vi "testAo8b.vi"() -> ()   [LabVIEW 2011, in "run.lvlib"]
uses:
  Hal/testing/run.lvlib
  <vilib>/Utility/error.llb/DialogType.ctl
  <vilib>/DAQmx/write.llb/DAQmx Write (Analog 2D DBL NChan NSamp).vi
  <vilib>/DAQmx/create/channels.llb/DAQmx Create Channel (AO-Voltage-Basic).vi
  <vilib>/DAQmx/configure/timing.llb/DAQmx Timing (Sample Clock).vi
  <vilib>/DAQmx/miscellaneous.llb/DAQmx Fill In Error Info.vi
  Program Files/National Instruments/LabVIEW 2011/resource/objmgr/daqmx.rc
panel:
  out "CurrWritePos":dbl
  out "TotalSampPerChanGenerated":dbl
  out "number of samples written per channel":u32
  in  "Clock Source":tag="/Ao8b/PFI8"
  in  "stop":bool
  in  "Data":dbl[][](array[numeric])=[[0.0, -0.00465, -0.00465, -0.00465, -0.00465, -0.00465, -0.00465, -0.00423429, -0.00423429, -0.00423429, -0.00423429, -0.00423429, -0.00381858, -0.00381858, -0.00381858, -0.00381858, -0.00381858, -0.00381858, -0.0034028699999999997, -0.0034028699999999997, -0.0034028699999999997, -0.0034028699999999997, -0.0034028699999999997, -0.00298716, -0.00298716, -0.00298716, -0.00298716, -0.00298716, -0.00298716, -0.00257145, -0.00257145, -0.00257145, -0.00257145, -0.0021557399999999997, -0.0021557399999999997, -0.0021557399999999997, -0.0021557399999999997, -0.0021557399999999997, -0.0021557399999999997, -0.00174003, -0.00174003, -0.00174003, -0.00174003, -0.00174003, -0.00132432, -0.00132432, -0.00132432, -0.00132432, -0.00132432, -0.00132432, -0.0009086099999999998, -0.0009086099999999998, -0.0009086099999999998, -0.0009086099999999998, -0.0009086099999999998, -0.0004929000000000001, -0.0004929000000000001, -0.0004929000000000001, -0.0004929000000000001, -0.0004929000000000001, -0.0004929000000000001, -0.0004929000000000001, -0.0004929000000000001], [0.0, -0.01554, -0.01554, -0.01554, -0.0151700148, -0.0151700148, -0.0151700148, -0.0151700148, -0.0148000296, -0.0148000296, -0.0148000296, -0.0144300444, -0.0144300444, -0.0144300444, -0.014060059199999999, -0.014060059199999999, -0.014060059199999999, -0.014060059199999999, -0.014060059199999999, -0.013690074, -0.013690074, -0.0133200888, -0.0133200888, -0.0133200888, -0.0133200888, -0.012950103599999999, -0.012950103599999999, -0.012950103599999999, -0.0125801184, -0.0125801184, -0.0125801184, -0.0122101332, -0.0122101332, -0.0122101332, -0.011840148, -0.011840148, -0.011840148, -0.0114701628, -0.0114701628, -0.0114701628, -0.0114701628, -0.0111001776, -0.0111001776, -0.0107301924, -0.0107301924, -0.0107301924, -0.0107301924, -0.0107301924, -0.010360207199999999, -0.010360207199999999, -0.010360207199999999, -0.009990222, -0.009990222, -0.009990222, -0.0096202368, -0.0096202368, -0.0096202368, -0.0096202368, -0.009250251599999999, -0.009250251599999999, -0.0088802664, 0.0, 0.0], [0.0, -0.03996, -0.03996, -0.03996, -0.03996, -0.03996, -0.037739988, -0.037739988, -0.037739988, -0.037739988, -0.037739988, -0.035519976, -0.035519976, -0.035519976, -0.035519976, -0.035519976, -0.033299964, -0.033299964, -0.033299964, -0.033299964, -0.033299964, -0.031079952, -0.031079952, -0.031079952, -0.031079952, -0.031079952, -0.02885994, -0.02885994, -0.02885994, -0.02885994, -0.02885994, -0.026639928000000004, -0.026639928000000004, -0.026639928000000004, -0.026639928000000004, -0.026639928000000004, -0.024419916000000003, -0.024419916000000003, -0.024419916000000003, -0.024419916000000003, -0.024419916000000003, -0.022199904000000003, -0.022199904000000003, -0.022199904000000003, -0.022199904000000003, -0.022199904000000003, -0.019979892000000003, -0.019979892000000003, -0.019979892000000003, -0.019979892000000003, -0.019979892000000003, -0.017759880000000002, -0.017759880000000002, -0.017759880000000002, -0.017759880000000002, -0.017759880000000002, -0.015539868000000002, -0.015539868000000002, -0.015539868000000002, -0.015539868000000002, -0.015539868000000002, 0.0, 0.0], [0.0, -0.735, -0.735, -0.70673076, -0.70673076, -0.6784615199999999, -0.6784615199999999, -0.6784615199999999, -0.6784615199999999, -0.65019228, -0.62192304, -0.62192304, -0.62192304, -0.5936538, -0.5936538, -0.56538456, -0.56538456, -0.53711532, -0.53711532, -0.53711532, -0.50884608, -0.50884608, -0.48057684, -0.48057684, -0.4523076, -0.4523076, -0.4523076, -0.42403835999999995, -0.42403835999999995, -0.42403835999999995, -0.39576912, -0.36749988, -0.33923063999999997, -0.33923063999999997, -0.33923063999999997, -0.31096139999999994, -0.31096139999999994, -0.31096139999999994, -0.28269215999999997, -0.28269215999999997, -0.25442292, -0.25442292, -0.22615368000000002, -0.22615368000000002, -0.22615368000000002, -0.19788443999999994, -0.19788443999999994, -0.16961519999999997, -0.16961519999999997, -0.14134596, -0.14134596, -0.14134596, -0.11307671999999991, -0.08480747999999994, -0.08480747999999994, -0.08480747999999994, -0.08480747999999994, -0.05653823999999996, -0.05653823999999996, -0.02826899999999999, -0.02826899999999999, 0.0, 0.0]]
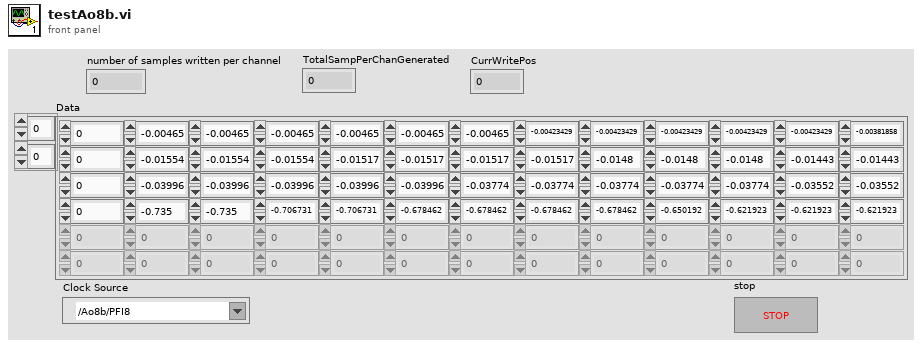
[diagram p1: front panel]
types:
  T1 = typedef "DialogType.ctl" = u16
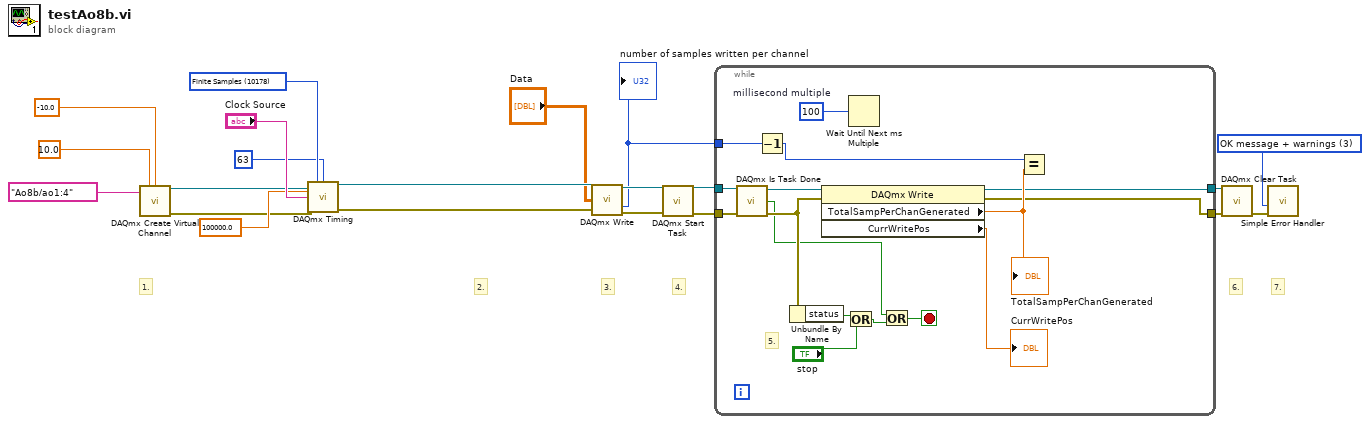
[diagram p0: block diagram]
diagram:
  w11 = T1 3 items=["no dialog", "OK message", "continue or stop message", "OK message + warnings", "continue/stop + warnings"] ("type of dialog (OK msg:1)")
  w19 = 10178 items=["Finite Samples"=10178, "Continuous Samples"=10123] ("sample mode")
  # "7."
  # "6."
  # "4."
  # "3."
  # "2."
  # "1."
  n1 = call-poly <vilib>:"DAQmx Create Virtual Channel.vi"("maximum value"=10.0 ("Maximum Value"), "minimum value"=-10.0 ("Minimum Value"), "physical channels"=tag "Ao8b/ao1:4" ("Physical Channels")) -> ("task out"=w3:refnum<k21>, "error out"=w2:errorcluster)  [unwired: 11 in]
  n2 = call-poly <vilib>:"DAQmx Timing.vi"("task/channels in"=w3, "sample mode"=w19, "samples per channel"=63, "rate"=100000.0 ("External Sample Clock Rate"), "source"="Clock Source", "error in"=w2) -> ("task out"=w13:refnum<k21>, "error out"=w8:errorcluster)  [unwired: 8 in]
  n3 = call-poly <vilib>:"DAQmx Write.vi"("task/channels in"=w13, "data"="Data", "error in"=w8) -> ("task out"=w16:refnum<k21>, "number of samples written per channel"=w4:u32, "error out"=w15:errorcluster)  [unwired: 10 in]
  "number of samples written per channel" <- w4
  n4 = call <vilib>:"DAQmx Start Task.vi"("task/channels in"=w16, "error in"=w15) -> ("task out"=w20:refnum<k21>, "error out"=w14:errorcluster)  [unwired: 12 in]
  n5 = while {
    tunnel: w20 -> [w37]
    tunnel: [w26] -> w10
    tunnel: w14 -> [w36]
    tunnel: [w27] -> w9
    tunnel: w4 -> [w31]
    stop <- w24 stop-if-true
    w34 = u32 100  # millisecond multiple
    # "5."
    n6 = call <vilib>:"DAQmx Is Task Done.vi"("task/channels in"=w37, "error in"=w36) -> ("task out"=w32:refnum<k21>, "task done?"=w22:bool, "error out"=w33:errorcluster)  [unwired: 11 in]
    n7 = Decrement(x=w31) -> (x-1=w30:u32)
    n8 = Unbundle By Name(w33) -> ("status"=w35:bool)
    n9 = property class="DAQmx Write"(reference=w32, error in=w33) -> (reference out=w26:refnum<k21>, error out=w27:errorcluster, "TotalSampPerChanGenerated"=w29:dbl, "CurrWritePos"=→"CurrWritePos":dbl)
    "TotalSampPerChanGenerated" <- w29
    n10 = Or(x=w35, y="stop") -> (x .or. y?=w23:bool)
    n11 = Wait Until Next ms Multiple(millisecond multiple=w34) -> ()  [unwired: 1 out]
    n12 = Or(x=w22, y=w23) -> (x .or. y?=w24:bool)
    n13 = Equal?(x=w30, y=w29) -> ()  [unwired: 1 out]
  }
  n14 = call <vilib>:"DAQmx Clear Task.vi"("task in"=w10, "error in"=w9) -> ("error out"=w21:errorcluster)  [unwired: 13 in]
  n15 = call <vilib>:"Simple Error Handler.vi"("type of dialog (OK msg:1)"=w11, "error in (no error)"=w21) -> ()  [unwired: 3 in, 5 out]
